vi "Create DAQ Chans.vi"(8 "error in (no error)":errorcluster, 11 "Device Reference":T1 format="%.0x") -> (0 "error out":errorcluster, 1 "SampleRate":dbl, 2 "task out":refnum<k21>, 3 "Device Reference out":T1 format="%.0x")   [LabVIEW 2011, in "PXIe-433x Custom Device.lvlib"]
uses:
  PXIe-433x Custom Device.lvlib
  <vilib>/NI Veristand/Custom Device API/Custom Device Item Ref.ctl
  <vilib>/NI Veristand/Custom Device Tools/Custom Device Utility Library/NI VeriStand - Search for All Items by GUID.vi
  <vilib>/NI Veristand/Custom Device API/Get Item Property (Double).vi
  Global.vi
  <vilib>/NI Veristand/Custom Device API/Custom Device API.lvlib
  <vilib>/NI Veristand/Custom Device Tools/Custom Device Utility Library/Custom Device Utility Library.lvlib
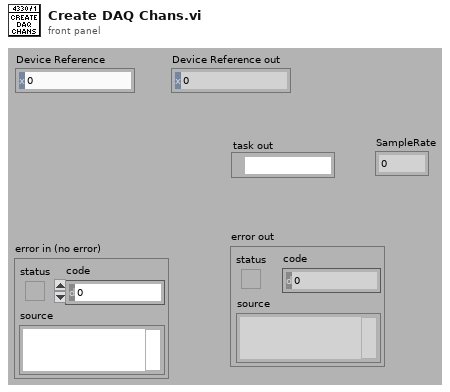
[diagram p1: front panel]
types:
  T1 = typedef "Custom Device API.lvlib/Custom Device Item Ref.ctl" = u64
  T2 = cluster{"Channel FIFO Buffer Index":u64, "Section Ref in":T1}[]
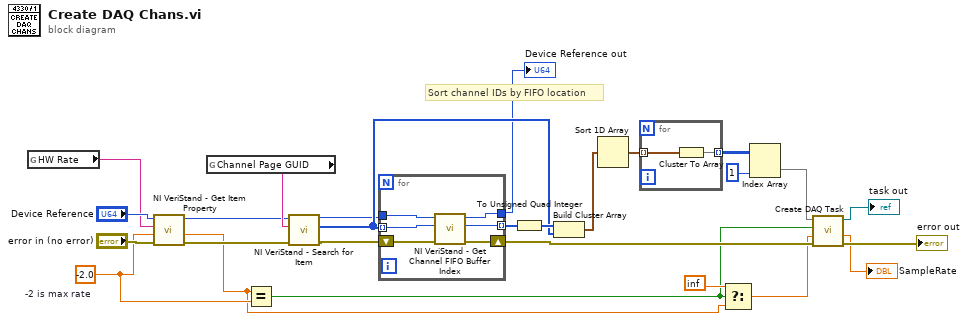
[diagram p0: block diagram]
diagram:
  w5 = -2.0  # -2 is max rate
  # "Sort channel IDs by FIFO location"
  n1 = global read "Global.vi" "HW Rate"() -> (w6:string)
  n2 = call-poly <vilib>:"NI VeriStand - Get Item Property.vi"("error in (no error)"="error in (no error)", "Default Value"=w5, "Property Name"=w6, "Item Ref in"="Device Reference") -> ("error out"=w7:errorcluster, "Value"=w1:dbl, "Item Ref out"=w8:T1)  [unwired: 4 in, 1 out]
  n3 = global read "Global.vi" "Channel Page GUID"() -> (w14:string)
  n4 = Equal?(x=w1, y=w5) -> (x = y?=w2:bool)
  n5 = call-poly <vilib>:"NI VeriStand - Search for Item.vi"("error in"=w7, "Item GUID"=w14, "Section Ref in"=w8) -> ("error out"=w17:errorcluster, "Item Refs"=w16:T1[], "Section Ref out"=w15:T1)  [unwired: 5 in, 1 out]
  n6 = for {
    tunnel: w16 -> [w32] mode=indexing
    tunnel: w15 -> [w31]
    shift-right: [w28] -> w12
    shift-left: w17 -> [w30]
    tunnel: [w29] -> w22 mode=indexing
    tunnel: [w27] -> w13
    n7 = call <vilib>:"NI VeriStand - Get Channel FIFO Buffer Index.vi"("error in"=w30, "Channel Ref"=w32, "Device Ref in"=w31) -> ("error out"=w28:errorcluster, "Channel FIFO Buffer Index"=w29:i32, "Device Ref out"=w27:T1)  [unwired: 4 in, 2 out]
  }
  "Device Reference out" <- w13
  n8 = To Unsigned Quad Integer(1:w22) -> (0:w21:u64[])
  n9 = Build Cluster Array ("Index & Bundle Cluster Array")(w21, w16) -> (w23:T2)
  n10 = Sort 1D Array(array=w23) -> (sorted array=w24:T2)
  n11 = for {
    tunnel: w24 -> [w33] mode=indexing
    tunnel: [w34] -> w20 mode=indexing
    n12 = Cluster To Array(cluster=w33) -> (array=w34:T1[])
  }
  n13 = Select(t=inf, s=w2, f=w1) -> (s? t:f=w3:dbl)
  n14 = Index Array(array=w20, index (col)=1 ("disabled index (col)")) -> (element=w18:T1[])  [unwired: 1 in]
  n15 = call "Create DAQ Task.vi"("error in"=w12, "User provided rate"=w3, "Search for Max rate? (F)"=w2, "Channels"=w18) -> ("error out"=→"error out":errorcluster, "Actual rate"=→"SampleRate":dbl, "task out"=→"task out":refnum<k21>)  [unwired: 5 in]
